vi "File_Start.vi"(8 "error in":errorcluster, 9 "Path":path, 10 "Name":string, 11 "File.lvclass (IN)":refnum<class "File.lvclass">) -> (0 "error out":errorcluster, 3 "File.lvclass (OUT)":refnum<class "File.lvclass">)   [LabVIEW 2013, in "File.lvclass"]
uses:
  File.lvclass
  File.lvclass/File.ctl
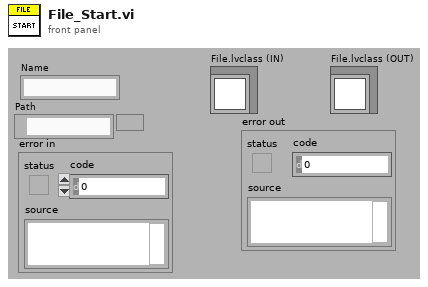
[diagram p1: front panel]
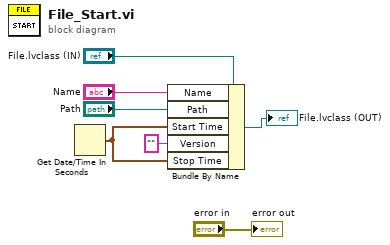
[diagram p0: block diagram]
diagram:
  n1 = Get Date/Time In Seconds() -> (seconds since 1Jan1904=w3:timestamp)
  n2 = Bundle By Name(cluster="File.lvclass (IN)", "Name"="Name", "Path"="Path", "Start Time"=w3, "Version"="", "Stop Time"=w3) -> (→"File.lvclass (OUT)":refnum<class "File.lvclass">)
  "error out" <- "error in"
